vi "CRYClose StepRefs.vi"   [LabVIEW 2013]
uses:
  CRYSystem/Program/CRYRef nums global.vi
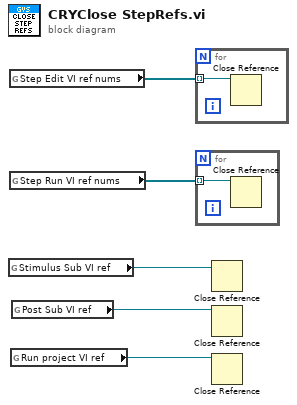
[diagram p0: block diagram]
diagram:
  n1 = global read "CRYRef nums global.vi" "Stimulus Sub VI ref"() -> (w5:refnum<vi>)
  n2 = global read "CRYRef nums global.vi" "Step Edit VI ref nums"() -> (w2:refnum<vi>[])
  n3 = global read "CRYRef nums global.vi" "Step Run VI ref nums"() -> (w1:refnum<vi>[])
  n4 = global read "CRYRef nums global.vi" "Run project VI ref"() -> (w3:refnum<vi>)
  n5 = global read "CRYRef nums global.vi" "Post Sub VI ref"() -> (w4:refnum<vi>)
  n6 = for {
    tunnel: w2 -> [w6] mode=indexing
    n7 = Close Reference(reference=w6) -> ()  [unwired: 1 in, 1 out]
  }
  n8 = for {
    tunnel: w1 -> [w7] mode=indexing
    n9 = Close Reference(reference=w7) -> ()  [unwired: 1 in, 1 out]
  }
  n10 = Close Reference(reference=w5) -> ()  [unwired: 1 in, 1 out]
  n11 = Close Reference(reference=w4) -> ()  [unwired: 1 in, 1 out]
  n12 = Close Reference(reference=w3) -> ()  [unwired: 1 in, 1 out]
